vi "SelectData.vi"(8 "error in (no error)":errorcluster, 10 "Condition Data":variant[](array[variant]), 11 "object in":refnum<class "TableLogger_SQLite_Actor.lvclass">) -> (0 "error out":errorcluster, 2 "Data Clusters":variant[](array[variant]), 3 "object out":refnum<class "TableLogger_SQLite_Actor.lvclass">)   [LabVIEW 2015, in "TableLogger_SQLite_Actor.lvlib" / "TableLogger_SQLite_Actor.lvclass"]
uses:
  TableLogger_SQLite_Actor.lvclass
  TableLogger_SQLite_Actor.lvclass/TableLogger_SQLite_Actor.ctl
panel:
  # "Connector Pane"
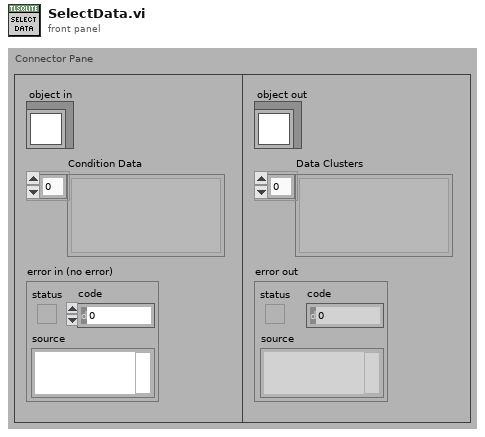
[diagram p1: front panel]
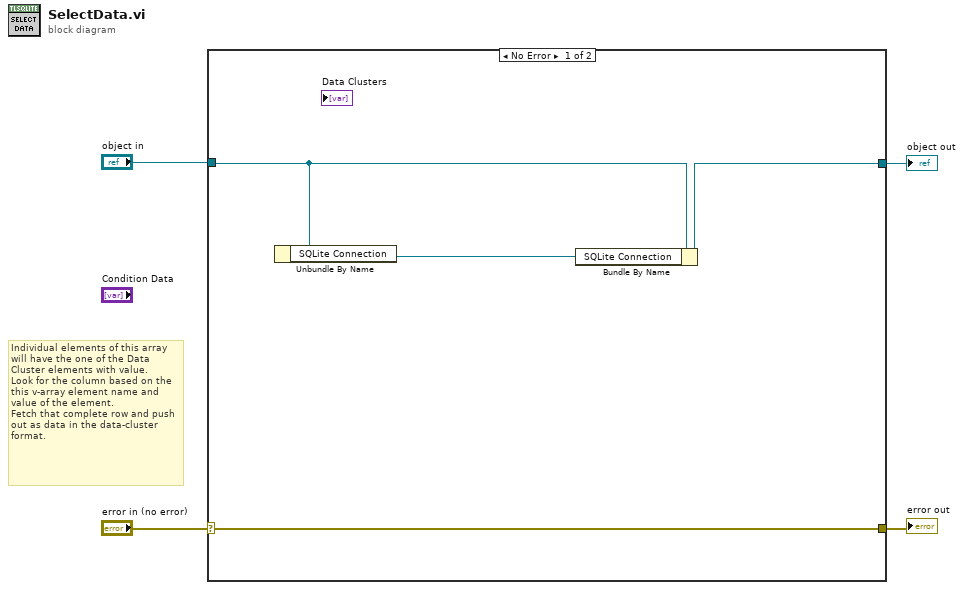
[diagram p0: block diagram]
diagram:
  # "Individual elements of this array will have the one of the Data Cluster elements with value.\nLook for the column based on the this v-array element name and value of the element.\nFetch that complete row and push out as data in the data-cluster format."
  n1 = case shown="No Error" "error in (no error)" {
    selector: "error in (no error)" -> [w7 w10]
    tunnel: [w7 w10] -> w3
    tunnel: [w5 w9] -> w1
    tunnel: "object in" -> [w6 w9]
    frame No Error {
      n2 = Unbundle By Name(w6) -> ("SQLite Connection"=w8:refnum<class "Connection.lvclass">)
      n3 = Bundle By Name(cluster=w6, "SQLite Connection"=w8) -> (w5:refnum<class "TableLogger_SQLite_Actor.lvclass">)
    }
    frame Error {
    }
  }
  "error out" <- w3
  "object out" <- w1
